vi "Example Simple - Bits.vi"(11 "character":string) -> (3 "bits":u8)   [LabVIEW 2013]
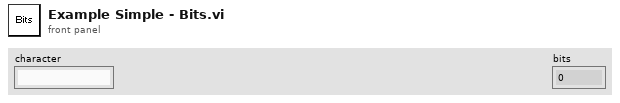
[diagram p1: front panel]
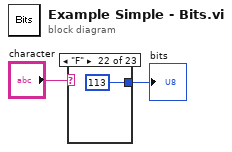
[diagram p0: block diagram]
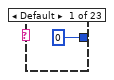
[diagram p2: hidden frame]
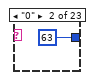
[diagram p3: hidden frame]
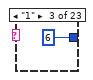
[diagram p4: hidden frame]
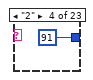
[diagram p5: hidden frame]
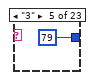
[diagram p6: hidden frame]
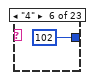
[diagram p7: hidden frame]
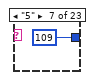
[diagram p8: hidden frame]
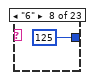
[diagram p9: hidden frame]
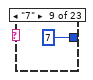
[diagram p10: hidden frame]
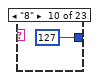
[diagram p11: hidden frame]
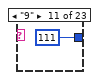
[diagram p12: hidden frame]
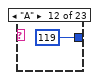
[diagram p13: hidden frame]
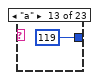
[diagram p14: hidden frame]
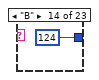
[diagram p15: hidden frame]
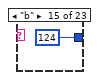
[diagram p16: hidden frame]
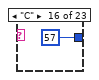
[diagram p17: hidden frame]
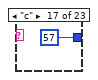
[diagram p18: hidden frame]
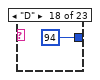
[diagram p19: hidden frame]
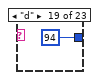
[diagram p20: hidden frame]
diagram:
  n1 = case shown="\"F\"" "character" {
    tunnel: [u8 0 u8 63 u8 6 u8 91 u8 79 u8 102 u8 109 u8 125 u8 7 u8 127 u8 111 u8 119 u8 119 u8 124 u8 124 u8 57 u8 57 u8 94 u8 94 u8 121 u8 121 u8 113 u8 113] -> w1
    frame Default {
    }
    frame "0" {
    }
    frame "1" {
    }
    frame "2" {
    }
    frame "3" {
    }
    frame "4" {
    }
    frame "5" {
    }
    frame "6" {
    }
    frame "7" {
    }
    frame "8" {
    }
    frame "9" {
    }
    frame "A" {
    }
    frame "a" {
    }
    frame "B" {
    }
    frame "b" {
    }
    frame "C" {
    }
    frame "c" {
    }
    frame "D" {
    }
    frame "d" {
    }
    frame "E" {
    }
    frame "e" {
    }
    frame "F" {
    }
    frame "f" {
    }
  }
  "bits" <- w1
